vi "rdb_json_decode_number.vi"(8 "error in (no error)":errorcluster, 9 "offset (0)":i32, 11 "json":string) -> (0 "error out":errorcluster, 1 "offset past match":i32, 2 "value":variant, 3 "type":T1)   [LabVIEW 2017]
uses:
  rdb_json_type.ctl
  <vilib>/Utility/error.llb/Error Cluster From Error Code.vi
  <vilib>/regexp/Match Regular Expression.xnode
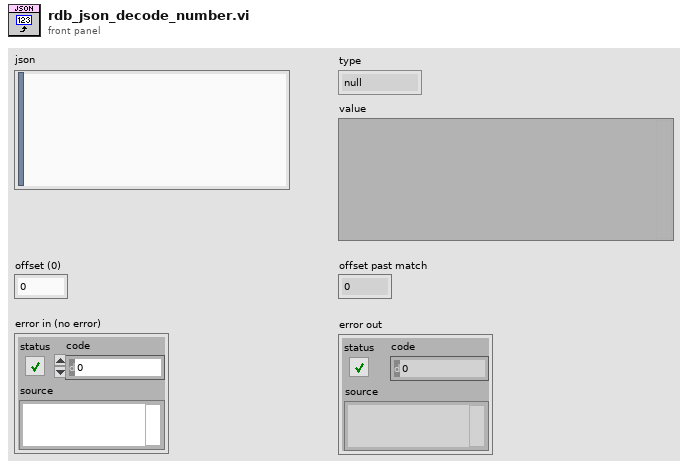
[diagram p1: front panel]
types:
  T1 = typedef "rdb_json_type.ctl" = enum8{"null", "bool", "int", "uint", "float", "string", "array", "object", "invalid"}
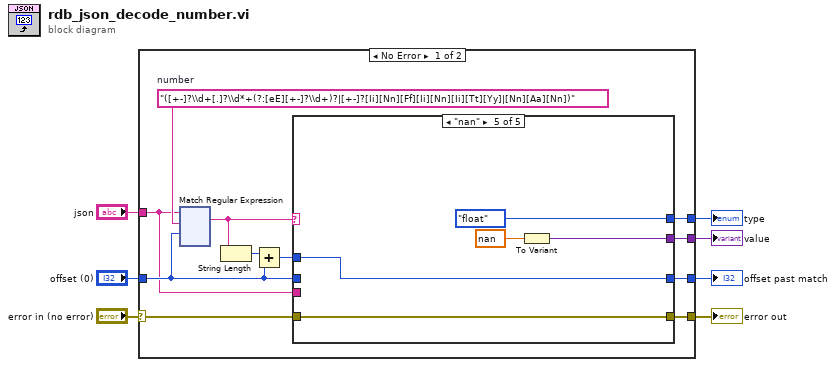
[diagram p0: block diagram]
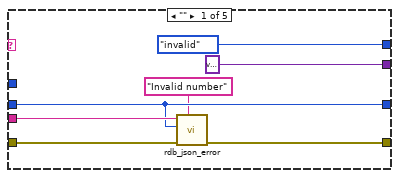
[diagram p2: hidden frame]
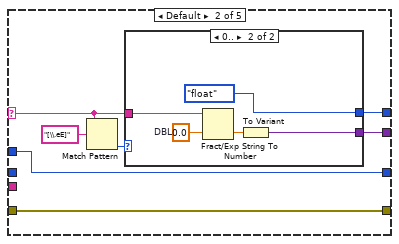
[diagram p3: hidden frame]
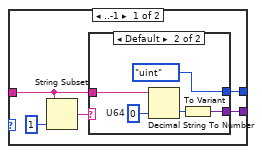
[diagram p4: hidden frame]
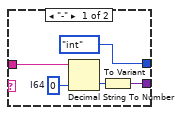
[diagram p5: hidden frame]
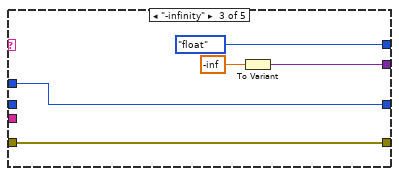
[diagram p6: hidden frame]
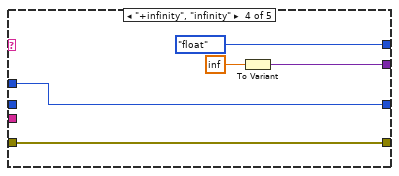
[diagram p7: hidden frame]
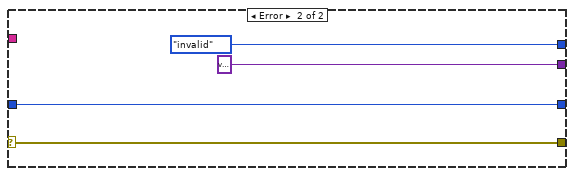
[diagram p8: hidden frame]
diagram:
  n1 = case shown="No Error" "error in (no error)" {
    selector: "error in (no error)" -> [w17 w185]
    tunnel: "json" -> [w8 _]
    tunnel: [w18 w185] -> w6
    tunnel: "offset (0)" -> [w11 w184]
    tunnel: [w16 w184] -> w3
    tunnel: [w15 rdb_json_type."invalid" ("type")] -> w2
    tunnel: [w14 variant ("Variant")] -> w1
    frame No Error {
      w10 = "([+-]?\\d+[.]?\\d*+(?:[eE][+-]?\\d+)?|[+-]?[Ii][Nn][Ff][Ii][Nn][Ii][Tt][Yy]|[Nn][Aa][Nn])"  # number
      n2 = xnode "Match Regular Expression"("input string"=w8, "regular expression"=w10, "offset (0)"=w11) -> ("whole match"=w9:string)  [unwired: 3 in, 4 out]
      n3 = String Length(string=w9) -> (length=w13:i32)
      n4 = Add(x=w13, y=w11) -> (x+y=w12:i32)
      n5 = case shown="\"nan\"" w9 {
        selector: w9 -> [_ w144 _ _ _]
        tunnel: w11 -> [w135 _ _ _ _]
        tunnel: [w134 w141 w171 w176 w181] -> w18
        tunnel: w17 -> [w137 w141 w171 w176 w181]
        tunnel: [w135 w140 w168 w173 w177] -> w16
        tunnel: [rdb_json_type."invalid" ("type") w143 rdb_json_type."float" ("type") rdb_json_type."float" ("type") rdb_json_type."float" ("type")] -> w15
        tunnel: [variant ("Variant") w142 w170 w175 w178] -> w14
        tunnel: w12 -> [_ w140 w168 w173 w177]
        tunnel: w8 -> [w136 _ _ _ _]
        frame "" {
          n6 = call "rdb_json_error.vi"("message"="Invalid number" ("error message (\"\")"), "error in (no error)"=w137, "offset (0)"=w135, "json"=w136) -> ("error out"=w134:errorcluster)  [unwired: 7 in]
        }
        frame Default {
          n7 = Match Pattern(string=w144, regular expression="[\\.eE]") -> (offset past match=w145:i32)  [unwired: 1 in, 3 out]
          n8 = case shown="0.." w145 {
            tunnel: w144 -> [w150 w166]
            tunnel: [w149 w163] -> w142
            tunnel: [w147 rdb_json_type."float" ("type")] -> w143
            frame ..-1 {
              n9 = String Subset(string=w150, length (rest)=1 ("length (rest)")) -> (substring=w148:string)  [unwired: 1 in]
              n10 = case shown="Default" w148 {
                tunnel: w150 -> [w156 w161]
                tunnel: [w153 w158] -> w149
                tunnel: [rdb_json_type."int" ("type") rdb_json_type."uint" ("type")] -> w147
                frame "-" {
                  w155 = i64 0  # I64
                  n11 = Decimal String To Number(string=w156, default (0L)=w155) -> (number=w154:i64)  [unwired: 1 in, 1 out]
                  n12 = To Variant(anything=w154) -> (Variant=w153:variant)
                }
                frame Default {
                  w160 = u64 0  # U64
                  n13 = Decimal String To Number(string=w161, default (0L)=w160) -> (number=w159:u64)  [unwired: 1 in, 1 out]
                  n14 = To Variant(anything=w159) -> (Variant=w158:variant)
                }
              }
            }
            frame 0.. {
              w165 = 0.0  # DBL
              n15 = Fract/Exp String To Number(string=w166, default (0 dbl)=w165) -> (number=w164:dbl)  [unwired: 2 in, 1 out]
              n16 = To Variant(anything=w164) -> (Variant=w163:variant)
            }
          }
        }
        frame "-infinity" {
          n17 = To Variant(anything=-inf) -> (Variant=w170:variant)
        }
        frame "+infinity", "infinity" {
          n18 = To Variant(anything=inf) -> (Variant=w175:variant)
        }
        frame "nan" {
          n19 = To Variant(anything=nan) -> (Variant=w178:variant)
        }
      }
    }
    frame Error {
    }
  }
  "error out" <- w6
  "offset past match" <- w3
  "type" <- w2
  "value" <- w1
